vi "Flywheel_Logic_TESTING.vi"() -> ()   [LabVIEW 2019]
panel:
  in  "search_value":ext
  in  "array":dbl[][](array[numeric])=[[40.0, 5800.0], [50.0, 5100.0], [70.0, 4900.0], [80.0, 4890.0], [130.0, 4750.0], [150.0, 4675.0], [180.0, 4650.0]]
  out "RPM output":dbl
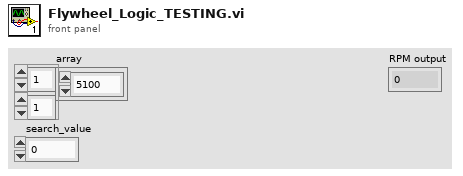
[diagram p1: front panel]
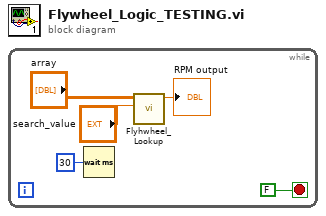
[diagram p0: block diagram]
diagram:
  n1 = while {
    stop <- FALSE stop-if-true
    n2 = Wait (ms)(milliseconds to wait=u32 30) -> ()  [unwired: 1 out]
    n3 = call "Flyhwheel_Lookup.vi"("search_value"="search_value", "array"="array") -> ("RPM output"=→"RPM output":dbl)  [unwired: 9 in]
  }
